vi "create SLM image from mask.vi"(9 "low image path":path, 10 "high image path":path, 11 "Mask":T1) -> (2 "Image Pixels (U8)":u8[][](array[numeric]), 3 "Final image":T1)   [LabVIEW 2025]
uses:
  <vilib>/vision/Image Controls.llb/IMAQ Image.ctl
  <vilib>/vision/NI_Vision_Development_Module.lvlib
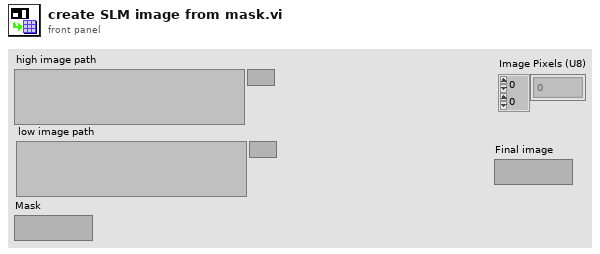
[diagram p1: front panel]
types:
  T1 = typedef "IMAQ Image.ctl" = refnum<image>
  T2 = typedef "Image Type" = u32
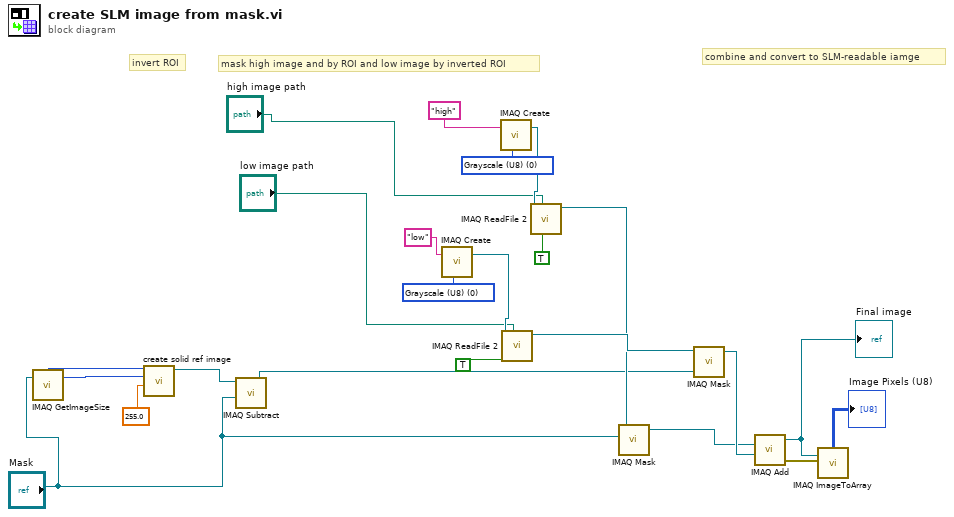
[diagram p0: block diagram]
diagram:
  w19 = T2 0 items=["Grayscale (U8)", "Grayscale (I16)", "Grayscale (SGL)", "Complex (CSG)", "RGB (U32)", "HSL (U32)", "RGB (U64)", "Grayscale (U16)"] ("Image Type")
  w23 = T2 0 items=["Grayscale (U8)", "Grayscale (I16)", "Grayscale (SGL)", "Complex (CSG)", "RGB (U32)", "HSL (U32)", "RGB (U64)", "Grayscale (U16)"] ("Image Type")
  # "combine and convert to SLM-readable iamge"
  # "mask high image and by ROI and low image by inverted ROI"
  # "invert ROI"
  n1 = call "IMAQ GetImageSize"("Image"="Mask") -> ("Y Resolution"=w4:i32, "X Resolution"=w5:i32)  [unwired: 3 in, 1 out]
  n2 = call "create solid ref image.vi"("Pixel Value (default 255)"=sgl 255.0, "Y resolution"=w4, "X resolution"=w5) -> ("solid image"=w9:T1)  [unwired: 7 in, 1 out]
  n3 = call "IMAQ Subtract"("Image Src A"=w9, "Image Src B"="Mask") -> ("Image Dst Out"=w12:T1)  [unwired: 5 in, 1 out]
  n4 = call "IMAQ Create"("Image Name"="low", "Image Type"=w19) -> ("New Image"=w18:T1)  [unwired: 3 in, 1 out]
  n5 = call "IMAQ Create"("Image Name"="high", "Image Type"=w23) -> ("New Image"=w22:T1)  [unwired: 3 in, 1 out]
  n6 = call "IMAQ ReadFile 2"("Use File Path Image Type"=TRUE, "File Path"="low image path", "Image"=w18) -> ("Image Out"=w15:T1)  [unwired: 4 in, 4 out]
  n7 = call "IMAQ ReadFile 2"("Use File Path Image Type"=TRUE, "File Path"="high image path", "Image"=w22) -> ("Image Out"=w14:T1)  [unwired: 4 in, 4 out]
  n8 = call "IMAQ Mask"("Image Mask"="Mask", "Image Src"=w14) -> ("Image Dst Out"=w11:T1)  [unwired: 3 in, 1 out]
  n9 = call "IMAQ Mask"("Image Mask"=w12, "Image Src"=w15) -> ("Image Dst Out"=w13:T1)  [unwired: 3 in, 1 out]
  n10 = call "IMAQ Add"("Image Src A"=w11, "Image Src B"=w13) -> ("Image Dst Out"=w1:T1, "error out"=w10:errorcluster)  [unwired: 5 in]
  "Final image" <- w1
  n11 = call "IMAQ ImageToArray"("error in (no error)"=w10, "Image"=w1) -> ("Image Pixels (U8)"=→"Image Pixels (U8)":u8[][])  [unwired: 2 in, 4 out]
